vi "Rec Get Column Properties (CR).vi"(4 "error in (no error)":errorcluster, 6 "column index":variant, 7 "command-recordset reference":T3) -> (0 "error out":errorcluster, 1 "column properties":T1, 3 "command-recordset reference out":T3)   [LabVIEW 2012, in "NI_Database_API_64.lvlib"]
doc: "Gets properties of the object as determined by the inputs. This VI works for connections, commands, recordsets, columns, and parameters. Wire data to the reference input to determine the polymorphic instance to use or manually select the instance."
uses:
  NI_Database_API_64.lvlib
  Command-Recordset.llb/Cmd-Rec Object Reference.ctl
  Rec Column Properties.ctl
  Auxilliary.llb/DB Tools DataTypes.ctl
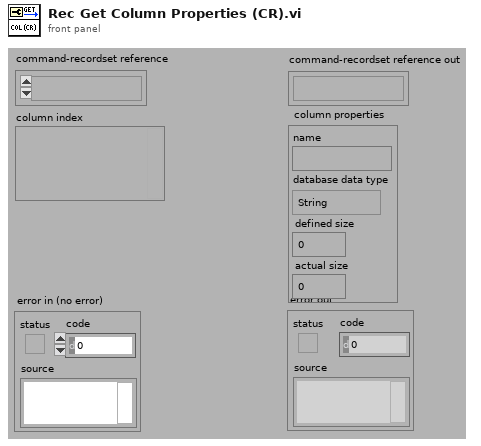
[diagram p1: front panel]
types:
  T1 = typedef "NI_Database_API_64.lvlib/Rec Column Properties.ctl" = cluster{"name":string, "database data type":T2, "defined size":i32, "actual size":i32}
  T2 = typedef "NI_Database_API_64.lvlib/DB Tools DataTypes.ctl" = enum16{"String", "Long (I32)", "Single (SGL)", "Double (DBL)", "Date/Time", "Binary"}
  T3 = typedef "NI_Database_API_64.lvlib/Cmd-Rec Object Reference.ctl" = refnum<k1>
  T4 = typedef "NI_Database_API_64.lvlib/Cmd-Rec Data Members.ctl" = cluster{"recordset reference":T5, "command reference":T6}
  T5 = typedef "NI_Database_API_64.lvlib/Rec ObjectReference.ctl" = refnum<k1>
  T6 = typedef "NI_Database_API_64.lvlib/Cmd ObjectReference.ctl" = refnum<k1>
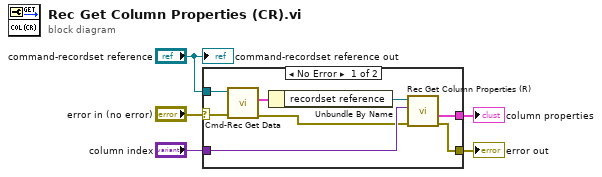
[diagram p0: block diagram]
diagram:
  n1 = case shown="No Error" "error in (no error)" {
    selector: "error in (no error)" -> [w6 w14]
    tunnel: [w13 w14] -> w5
    tunnel: "column index" -> [w12 _]
    tunnel: [w11 _] -> w3
    tunnel: "command-recordset reference" -> [w7 _]
    frame No Error {
      n2 = call "Cmd-Rec Get Data.vi"("error in (no error)"=w6, "command-recordset reference"=w7) -> ("error out"=w8:errorcluster, "data"=w9:T4)  [unwired: 2 in, 2 out]
      n3 = Unbundle By Name(w9) -> ("recordset reference"=w10:T5)
      n4 = call "Rec Get Column Properties (R).vi"("error in (no error)"=w8, "column index"=w12, "recordset reference"=w10) -> ("error out"=w13:errorcluster, "column properties"=w11:T1)  [unwired: 2 in, 1 out]
    }
    frame Error {
    }
  }
  "error out" <- w5
  "column properties" <- w3
  "command-recordset reference out" <- "command-recordset reference"
